vi "vince yopo.vi"(11 "Input Value":bool) -> (3 "Yopo'd value":bool)   [LabVIEW 2019]
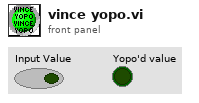
[diagram p1: front panel]
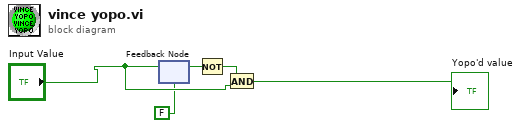
[diagram p0: block diagram]
diagram:
  n1 = feedback #1(FALSE) -> (w2:bool)
  n2 = feedback-in #1("Input Value") -> ()
  n3 = Not(x=w2) -> (.not. x?=w3:bool)
  n4 = And(x=w3, y="Input Value") -> (x .and. y?=→"Yopo'd value":bool)
